vi "hse-application_DetermineProgramVersion.vi"(8 "error in":errorcluster, 11 "Application in":refnum<class "hse-application.lvclass">) -> (0 "error out":errorcluster, 3 "Application out":refnum<class "hse-application.lvclass">)   [LabVIEW 2020, in "hse-application.lvclass"]
doc: "____\nHAMPEL SOFTWARE ENGINEERING v3.8.0 (2023-12-18 14:41)"
uses:
  hse-application.lvclass
  <vilib>/Utility/traverseref.llb/TRef TravTarget.ctl
  hse-application.lvclass/hse-application.ctl
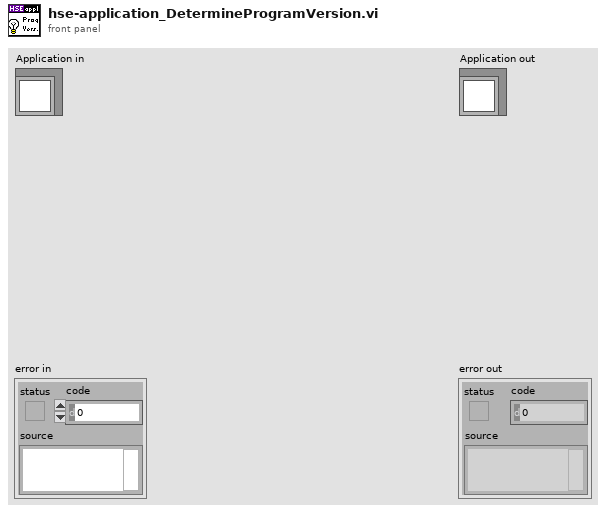
[diagram p1: front panel]
types:
  T1 = typedef "TRef TravTarget.ctl" = enum16{"FP", "BD", "Other"}
  T2 = enum32{"invalid app kind", "Development System", "Run Time System", "Student Edition", "Embedded LabVIEW", "Evaluation", "Custom"}
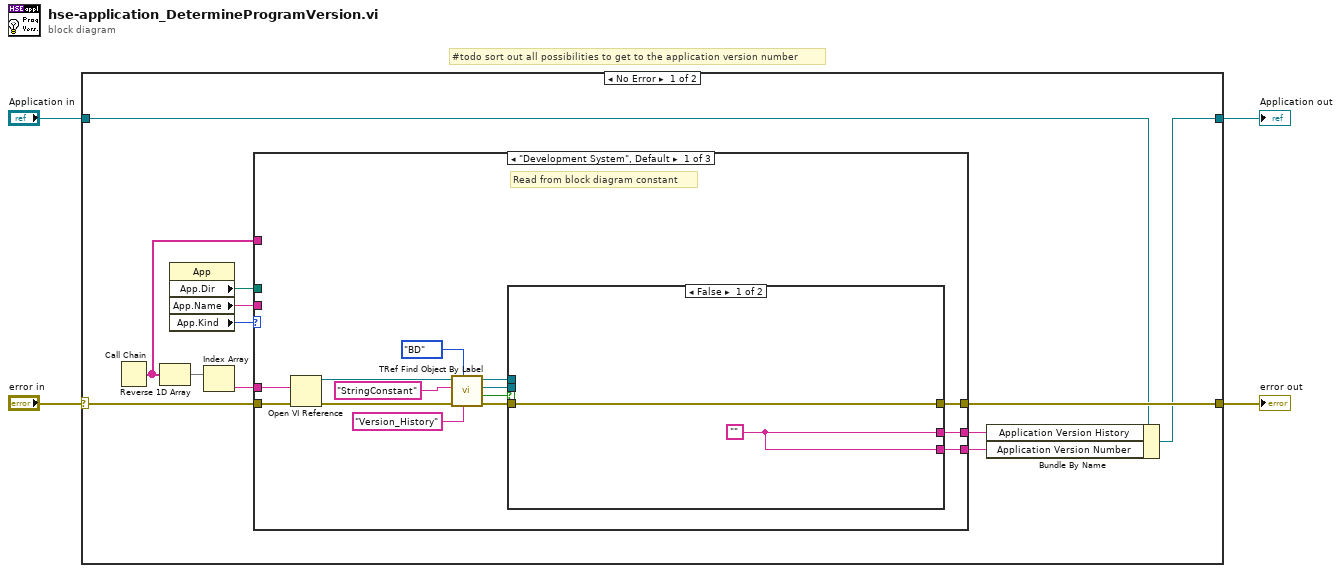
[diagram p0: block diagram]
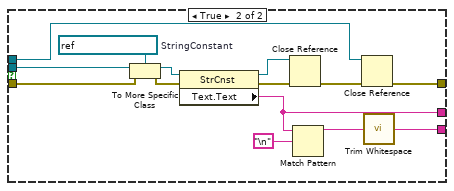
[diagram p2: hidden frame]
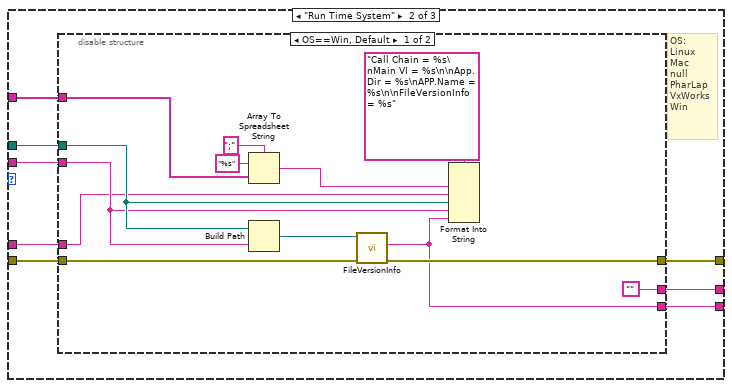
[diagram p3: hidden frame]
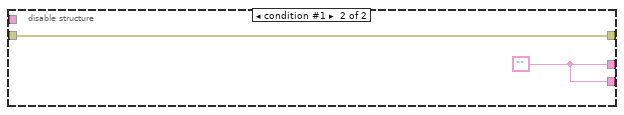
[diagram p4: hidden frame]
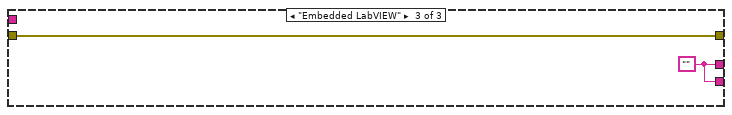
[diagram p5: hidden frame]
diagram:
  # "#todo sort out all possibilities to get to the application version number"
  n1 = case shown="No Error" "error in" {
    selector: "error in" -> [w14 w72]
    tunnel: [w15 w72] -> w3
    tunnel: [w8 w73] -> w1
    tunnel: "Application in" -> [w7 w73]
    frame No Error {
      n2 = Call Chain() -> (call chain=w9:string[])
      n3 = Reverse 1D Array(array=w9) -> (reversed array=w16:string[])
      n4 = property on="Property Node" class="App"() -> ("App.Dir"=w11:path, "App.Name"=w10:string, "App.Kind"=w6:T2)  [unwired: 2 in, 2 out]
      n5 = Index Array(array=w16) -> (element=w13:string)  [unwired: 1 in]
      n6 = case shown="\"Development System\", Default" w6 {
        tunnel: w14 -> [w21 w53 w71]
        tunnel: [w19 w52 w71] -> w15
        tunnel: w13 -> [w20 w54 _]
        tunnel: [w18 w51 w70] -> w5
        tunnel: [w17 w50 w70] -> w12
        tunnel: w11 -> [_ w49 _]
        tunnel: w10 -> [_ w48 _]
        tunnel: w9 -> [_ w47 _]
        frame "Development System", Default {
          # "Read from block diagram constant"
          n7 = Open VI Reference(vi path=w20, error in (no error)=w21) -> (vi reference=w23:refnum<vi>, error out=w22:errorcluster)  [unwired: 4 in]
          n8 = call <vilib>:"TRef Find Object By Label.vi"("Label"="Version_History", "Traverse Target"=TRef_TravTarget."BD", "error in (no error)"=w22, "Class Name"="StringConstant", "VI Ref"=w23) -> ("error out"=w27:errorcluster, "Found?"=w28:bool, "Found Obj Ref"=w29:refnum<vi>, "dup VI Ref"=w30:refnum<vi>)  [unwired: 3 in]
          n9 = case shown="False" w28 {
            tunnel: w29 -> [_ w43]
            tunnel: w27 -> [w32 w42]
            tunnel: [w32 w34] -> w19
            tunnel: [w31 w37] -> w18
            tunnel: [w31 w36] -> w17
            tunnel: w30 -> [_ w33]
            frame False {
              w31 = "" ("Text.Text")
            }
            frame True {
              w44 = refnum<vi> refnum  # StringConstant
              n10 = To More Specific Class(target class=w44, reference=w43, error in=w42) -> (specific class reference=w45:refnum<vi>, error out=w46:errorcluster)
              n11 = property on="Property Node" class="StrCnst"(reference=w45, error in=w46) -> (reference out=w39:refnum<vi>, error out=w38:errorcluster, "Text.Text"=w37:string)
              n12 = Close Reference(reference=w39, error in (no error)=w38) -> (error out=w35:errorcluster)
              n13 = Match Pattern(string=w37, regular expression="\n" ("Line Feed Constant")) -> (before substring=w40:string)  [unwired: 1 in, 3 out]
              n14 = Close Reference(reference=w33, error in (no error)=w35) -> (error out=w34:errorcluster)
              n15 = call <vilib>:"Trim Whitespace.vi"("string"=w40) -> ("trimmed string"=w36:string)  [unwired: 1 in]
            }
          }
        }
        frame "Run Time System" {
          # "OS:\nLinux\nMac\nnull\nPharLap\nVxWorks\nWin"
          n16 = disable-structure "Conditional Disable Structure" shown="OS==Win, Default" {
            disable-tunnel: ["" ("Empty String Constant") w68] -> w51
            disable-tunnel: w54 -> [w56 _]
            disable-tunnel: w53 -> [w66 w69]
            disable-tunnel: [w65 w69] -> w52
            disable-tunnel: [w55 w68] -> w50
            disable-tunnel: w49 -> [w59 _]
            disable-tunnel: w48 -> [w58 _]
            disable-tunnel: w47 -> [w57 _]
            frame condition #0 (active) {
              n17 = Array To Spreadsheet String(delimiter (Tab)=";", array=w57, 3:"%s" ("format string")) -> (spreadsheet string=w61:string)
              n18 = Build Path(base path=w59, name or relative path=w58) -> (appended path=w64:path)
              n19 = call <vilib>:"FileVersionInfo.vi"("error in (no error)"=w66, "Application Path in"=w64) -> ("error out"=w65:errorcluster, "File Version Info"=w55:string)  [unwired: 6 in, 2 out]
              n20 = Format Into String(format string="Call Chain = %s\nMain VI = %s\n\nApp.Dir = %s\nAPP.Name = %s\n\nFileVersionInfo = %s", w61, w56, w59, w58, w55) -> ()  [unwired: 2 in, 2 out]
            }
            frame condition #1 {
              w68 = "" ("Empty String Constant")
            }
          }
        }
        frame "Embedded LabVIEW" {
          w70 = "" ("Empty String Constant")
        }
      }
      n21 = Bundle By Name(cluster=w7, "Application Version History"=w5, "Application Version Number"=w12) -> (w8:refnum<class "hse-application.lvclass">)
    }
    frame Error {
    }
  }
  "error out" <- w3
  "Application out" <- w1
